vi "Write ProgrammaticInitialization.vi"(8 "error in (no error)":errorcluster, 10 "ProgrammaticInitialization.lvclass":refnum<class "ProgrammaticInitialization.lvclass">, 11 "MiddlewareSALThisComponent in":refnum<class "MiddlewareSALThisComponent.lvclass">) -> (0 "error out":errorcluster, 3 "MiddlewareSALThisComponent out":refnum<class "MiddlewareSALThisComponent.lvclass">)   [LabVIEW 2016, in "MiddlewareSALThisComponent.lvclass"]
uses:
  MiddlewareSALThisComponent.lvclass
  ProgrammaticInitialization/ProgrammaticInitialization.lvclass
  MiddlewareSALThisComponent.lvclass/MiddlewareSALThisComponent.ctl
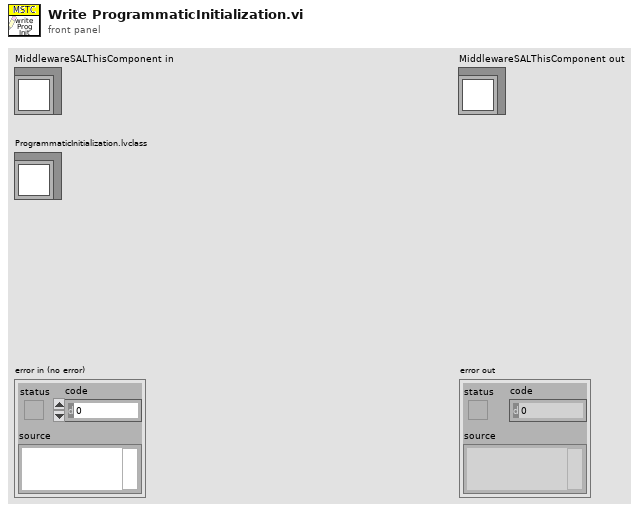
[diagram p1: front panel]
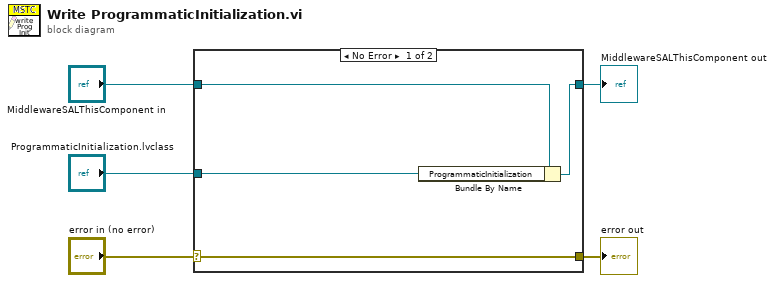
[diagram p0: block diagram]
diagram:
  n1 = case shown="No Error" "error in (no error)" {
    selector: "error in (no error)" -> [w9 w10]
    tunnel: [w9 w10] -> w4
    tunnel: [w7 w11] -> w2
    tunnel: "MiddlewareSALThisComponent in" -> [w8 w11]
    tunnel: "ProgrammaticInitialization.lvclass" -> [w6 _]
    frame No Error {
      n2 = Bundle By Name(cluster=w8, "ProgrammaticInitialization"=w6) -> (w7:refnum<class "MiddlewareSALThisComponent.lvclass">)
    }
    frame Error {
    }
  }
  "error out" <- w4
  "MiddlewareSALThisComponent out" <- w2
